vi "Handle Metric.vi"(8 "error in (no error)":errorcluster, 10 "Metric Update":T1, 11 "Volatus Core in":refnum<class "Volatus Core.lvclass">) -> (0 "error out":errorcluster, 3 "Volatus Core out":refnum<class "Volatus Core.lvclass">)   [LabVIEW 2020, in "Volatus.lvlib" / "Volatus Core.lvclass"]
uses:
  Volatus Core.lvclass
  Volatus Core.lvclass/Volatus Core.ctl
  Module/Module.lvclass
  C:/dev/lv20CE/relink/lv-volatus/Volatus/Module/Module.lvclass
  C:/dev/lv20CE/relink/lv-volatus/Volatus/Volatus Core/Volatus Core.lvclass
  Metric Update.ctl
  Volatus.lvlib
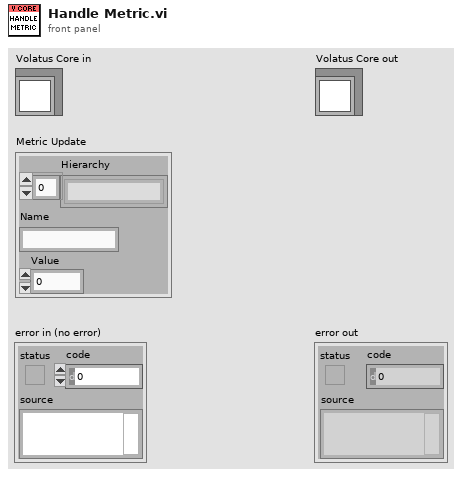
[diagram p1: front panel]
types:
  T1 = typedef "Volatus.lvlib/Metric Update.ctl" = cluster{"Hierarchy":string[], "Name":string, "Value":dbl}
  T2 = typedef "Volatus.lvlib/Module Status.ctl" = cluster{"Hierarchy":string[], "State":T3, "Substatus":map{string, string}, "Metrics":map{string, dbl}}
  T3 = typedef "Volatus.lvlib/Module.lvclass/State.ctl" = enum16{"Unknown", "Launched", "Starting", "Running", "Stopping", "Stopped", "Error - Starting", "Error - Run", "Error - Stopping"}
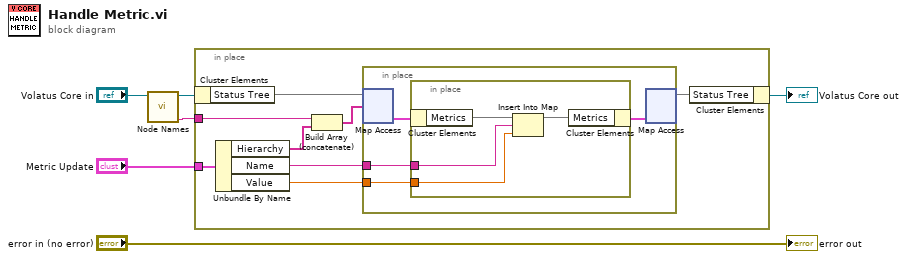
[diagram p0: block diagram]
diagram:
  n1 = call "Node Names.vi"("Module in"="Volatus Core in") -> ("Node"=w1:string, "Module out"=w2:refnum<class "Volatus Core.lvclass">)  [unwired: 6 in, 3 out]
  n2 = in-place {
    in-place-border: "Metric Update" -> [w14]
    in-place-border: w1 -> [w8]
    n3 = in-place-cluster #1(w2) -> ("Status Tree"=w13:map{string[], T2})
    n4 = Unbundle By Name(w14) -> ("Hierarchy"=w9:string[], "Name"=w12:string, "Value"=w11:dbl)
    n5 = Build Array (concatenate)(w8, w9) -> (w7:string[])
    n6 = in-place {
      in-place-border: w12 -> [w17]
      in-place-border: w11 -> [w16]
      n7 = in-place-map #2(w13, w7) -> (w18:T2)  [unwired: 1 in, 1 out]
      n8 = in-place {
        in-place-border: w17 -> [w21]
        in-place-border: w16 -> [w20]
        n9 = in-place-cluster #3(w18) -> ("Metrics"=w22:map{string, dbl})
        n10 = Insert Into Map(map in=w22, key=w21, value=w20) -> (map out=w19:map{string, dbl})  [unwired: 2 out]
        n11 = in-place-cluster #3("Metrics"=w19) -> (w15:T2)
      }
      n12 = in-place-map #2(w15) -> (w10:map{string[], T2})  [unwired: 1 in, 2 out]
    }
    n13 = in-place-cluster #1("Status Tree"=w10) -> (→"Volatus Core out":refnum<class "Volatus Core.lvclass">)
  }
  "error out" <- "error in (no error)"
